vi "RSNRPZ Sensor Self Test.vi"(8 "error in (no error)":errorcluster, 10 "Channel (1)":i32=1, 11 "VISA session":refnum<visa-resource-name> caption="VISA resource name") -> (0 "error out":errorcluster, 2 "Result":string, 3 "dup VISA session":refnum<visa-resource-name> caption="VISA resource name")   [LabVIEW 2010]
doc: "This VI performs a sensor test and returns a list of strings separated by commas. The contents of this test protocol is sensor-specific. For its meaning, please refer to the sensor documentation.\n\nRemote-control command(s):\nTEST:SENS?"
uses:
  rsnrpz_32.dll
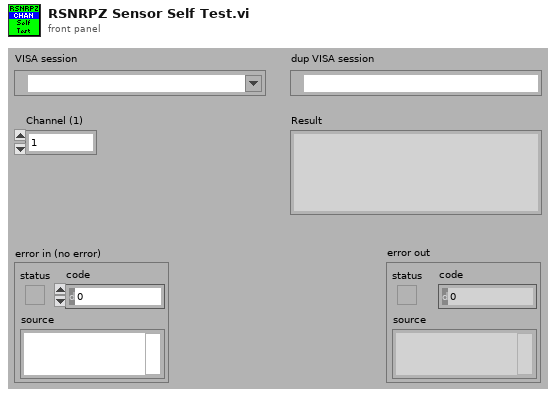
[diagram p1: front panel]
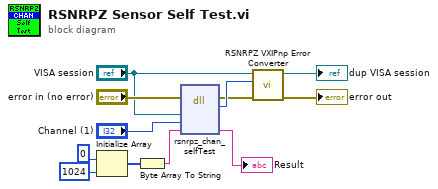
[diagram p0: block diagram]
diagram:
  n1 = Initialize Array(u8 0, 1024) -> (w10:u8[])
  n2 = Byte Array To String(unsigned byte array=w10) -> (string=w7:string)
  n3 = dll-call lib="rsnrpz_32.dll" fn="rsnrpz_chan_selfTest"(error in="error in (no error)", "VISA Session"="VISA session", "Channel"="Channel (1)", "Result"=w7) -> (error out=w5:errorcluster, "Status"=w9:i32, "Result"=→"Result":string)  [unwired: 4 in, 1 out]
  n4 = call <instrlib>:"RSNRPZ VXIPnp Error Converter.vi"("error in"=w5, "VXIPnp error code"=w9, "VISA session"="VISA session") -> ("error out"=→"error out":errorcluster, "dup VISA session"=→"dup VISA session":refnum<visa-resource-name>)  [unwired: 7 in]
